vi "ZLIB VI Tree__ogtk.vi"() -> ()   [LabVIEW 2014]
uses:
  <userlib>/_OpenG.lib/lvzip/lvzip.llb/ZLIB File Info Old__ogtk.ctl
  <userlib>/_OpenG.lib/lvzip/lvzip.llb/ZLIB Compress File Info__ogtk.ctl
  <userlib>/_OpenG.lib/lvzip/lvzip.llb/ZLIB Uncompress File Info__ogtk.ctl
  <userlib>/_OpenG.lib/lvzip/lvzip.llb/ZLIB Unzip Handle__ogtk.ctl
  <userlib>/_OpenG.lib/lvzip/lvzip.llb/ZLIB Zip Handle__ogtk.ctl
  <userlib>/_OpenG.lib/lvzip/lvzip.llb/ZLIB File Info__ogtk.ctl
  <userlib>/_OpenG.lib/lvzip/lvzip.llb/ZLIB Open Zip Archive__ogtk.vi
  <userlib>/_OpenG.lib/lvzip/lvzip.llb/ZLIB Open Unzip Archive__ogtk.vi
  <userlib>/_OpenG.lib/lvzip/lvzip.llb/ZLIB Store File__ogtk.vi
  <userlib>/_OpenG.lib/lvzip/lvzip.llb/ZLIB Extract File__ogtk.vi
  <userlib>/_OpenG.lib/lvzip/lvzip.llb/ZLIB Open Unzip Stream__ogtk.vi
  <userlib>/_OpenG.lib/lvzip/lvzip.llb/ZLIB Store Stream__ogtk.vi
  <userlib>/_OpenG.lib/lvzip/lvzip.llb/ZLIB Extract Stream__ogtk.vi
panel:
  out "file info":T1 {"file timestamp" format="%<%H:%M:%S\n%d/%m/%Y>T"; "external fa" format="%.0x"; "internal fa" format="%.0x"; "crc" format="%.0x"}
  in  "zip file handle":T2
  in  "unzip file handle":T3
  out "unzip file info internal":T4 {"external fa" format="%.0x"; "internal fa" format="%.0x"; "crc" format="%.0x"}
  out "zip file info internal":T5
  out "file info old":T6 {"file timestamp" format="%<%H:%M:%S\n%d/%m/%Y>T"; "external fa" format="%.0x"; "internal fa" format="%.0x"; "crc" format="%.0x"}
  # "ZIP file library using the open source zlib library code with extension from Gilles Vollant.\nIn order to create a multi platform LabVIEW VI library some minor modification have been\nmade to the zlib library and ZIP file extension. The exported functions are all declared as\n__cdecl since this is the only platform independant calling convention available on all\nLabVIEW platforms. Doing it in this way allows us to use only one VI library which imports\nthe according shared library module, instead of having to maintain different VI libraries\nonly for the sake of different calling conventions.\nBecause of this and in order to avoid any incompatibilities with existing zlib libraries the\nshared library module has also been renamed to lvzlib.dll/so/cfr."
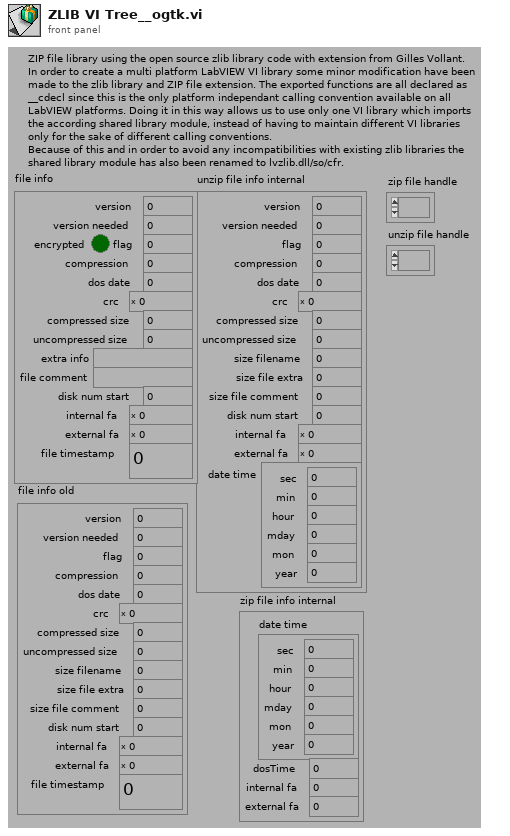
[diagram p1: front panel]
types:
  T1 = typedef "ZLIB File Info__ogtk.ctl" = cluster{"version":u32, "version needed":u32, "encrypted":bool, "flag":u32, "compression":i32, "dos date":u32, "crc":u32, "compressed size":u32, "uncompressed size":u32, "extra info":string, "file comment":string, "disk num start":u32, "internal fa":u32, "external fa":u32, "file timestamp":u32}
  T2 = typedef "ZLIB Zip Handle__ogtk.ctl" = refnum<k1>
  T3 = typedef "ZLIB Unzip Handle__ogtk.ctl" = refnum<k1>
  T4 = typedef "ZLIB Uncompress File Info__ogtk.ctl" = cluster{"version":u32, "version needed":u32, "flag":u32, "compression":u32, "dos date":u32, "crc":u32, "compressed size":u32, "uncompressed size":u32, "size filename":u32, "size file extra":u32, "size file comment":u32, "disk num start":u32, "internal fa":u32, "external fa":u32, "date time":cluster{"sec":i32, "min":i32, "hour":i32, "mday":i32, "mon":i32, "year":i32}}
  T5 = typedef "ZLIB Compress File Info__ogtk.ctl" = cluster{"date time":cluster{"sec":i32, "min":i32, "hour":i32, "mday":i32, "mon":i32, "year":i32}, "dosTime":u32, "internal fa":u32, "external fa":u32}
  T6 = typedef "ZLIB File Info Old__ogtk.ctl" = cluster{"version":u32, "version needed":u32, "flag":u32, "compression":u32, "dos date":u32, "crc":u32, "compressed size":u32, "uncompressed size":u32, "size filename":u32, "size file extra":u32, "size file comment":u32, "disk num start":u32, "internal fa":u32, "external fa":u32, "file timestamp":u32}
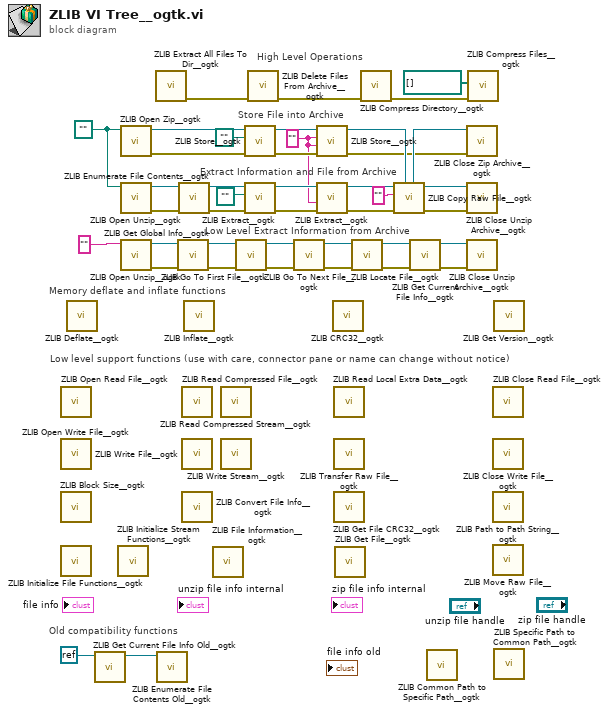
[diagram p0: block diagram]
diagram:
  w1 = ""
  w11 = path "" ("archive name")
  # "High Level Operations"
  # "Low level support functions (use with care, connector pane or name can change without notice)"
  # "Memory deflate and inflate functions"
  # "Old compatibility functions"
  # "Low Level Extract Information from Archive"
  # "Extract Information and File from Archive"
  # "Store File into Archive"
  n1 = call <userlib>:"ZLIB Open Read File__ogtk.vi"() -> ()  [unwired: 6 in, 4 out]
  n2 = call <userlib>:"ZLIB Open Write File__ogtk.vi"() -> ()  [unwired: 10 in, 2 out]
  n3 = call <userlib>:"ZLIB Block Size__ogtk.vi"() -> ()  [unwired: 2 in, 2 out]
  n4 = call <userlib>:"ZLIB Initialize File Functions__ogtk.vi"() -> ()  [unwired: 6 in, 2 out]
  n5 = call <userlib>:"ZLIB Deflate__ogtk.vi"() -> ()  [unwired: 5 in, 3 out]
  n6 = call <userlib>:"ZLIB Get Current File Info Old__ogtk.vi"("unzip Refnum"=refnum<k0> refnum) -> ("unzip Refnum out"=w21:T3)  [unwired: 3 in, 5 out]
  n7 = call <userlib>:"ZLIB Initialize Stream Functions__ogtk.vi"() -> ()  [unwired: 6 in, 2 out]
  n8 = call-poly <userlib>:"ZLIB Open Zip__ogtk.vi"("archive name"=w11) -> ("error out"=w30:errorcluster, "zip Refnum"=w31:T2)  [unwired: 4 in, 1 out]
  n9 = call-poly <userlib>:"ZLIB Open Unzip__ogtk.vi"("archive name"=w11) -> ("error out"=w23:errorcluster, "unzip Refnum"=w24:T3)  [unwired: 5 in]
  n10 = call-poly <userlib>:"ZLIB Open Unzip__ogtk.vi"("archive stream"="") -> ("error out"=w28:errorcluster, "unzip Refnum"=w29:T3)  [unwired: 5 in]
  n11 = call <userlib>:"ZLIB Extract All Files To Dir__ogtk.vi"() -> ("error out"=w18:errorcluster)  [unwired: 9 in, 2 out]
  n12 = call <userlib>:"ZLIB Enumerate File Contents Old__ogtk.vi"("unzip Refnum"=w21) -> ()  [unwired: 4 in, 7 out]
  n13 = call <userlib>:"ZLIB Get Global Info__ogtk.vi"("error in (no error)"=w28, "unzip Refnum"=w29) -> ("error out"=w34:errorcluster, "unzip Refnum out"=w35:T3)  [unwired: 2 in, 2 out]
  n14 = call <userlib>:"ZLIB Enumerate File Contents__ogtk.vi"("error in (no error)"=w23, "unzip Refnum"=w24) -> ("error out"=w26:errorcluster, "unzip Refnum out"=w27:T3)  [unwired: 5 in, 3 out]
  n15 = call <userlib>:"ZLIB Read Compressed File__ogtk.vi"() -> ()  [unwired: 8 in, 2 out]
  n16 = call <userlib>:"ZLIB Write File__ogtk.vi"() -> ()  [unwired: 7 in, 2 out]
  n17 = call <userlib>:"ZLIB Convert File Info__ogtk.vi"() -> ()  [unwired: 3 in, 1 out]
  n18 = call <userlib>:"ZLIB Inflate__ogtk.vi"() -> ()  [unwired: 5 in, 3 out]
  n19 = call <userlib>:"ZLIB File Information__ogtk.vi"() -> ()  [unwired: 4 in, 6 out]
  n20 = call <userlib>:"ZLIB Read Compressed Stream__ogtk.vi"() -> ()  [unwired: 7 in, 3 out]
  n21 = call <userlib>:"ZLIB Write Stream__ogtk.vi"() -> ()  [unwired: 7 in, 2 out]
  n22 = call <userlib>:"ZLIB Go To First File__ogtk.vi"("error in (no error)"=w34, "unzip Refnum"=w35) -> ("error out"=w40:errorcluster, "unzip Refnum out"=w41:T3)  [unwired: 4 in]
  n23 = call-poly <userlib>:"ZLIB Store__ogtk.vi"("error in (no error)"=w30, "source path"=path "", "zip Refnum"=w31) -> ("error out"=w5:errorcluster, "zip Refnum out"=w4:T2)  [unwired: 7 in]
  n24 = call-poly <userlib>:"ZLIB Extract__ogtk.vi"("error in (no error)"=w26, "target path"=path "", "unzip Refnum"=w27) -> ("error out"=w9:errorcluster, "unzip Refnum out"=w8:T3)  [unwired: 5 in]
  n25 = call <userlib>:"ZLIB Delete Files From Archive__ogtk.vi"("error in (no error)"=w18) -> ("error out"=w17:errorcluster)  [unwired: 9 in, 1 out]
  n26 = call <userlib>:"ZLIB Go To Next File__ogtk.vi"("error in (no error)"=w40, "unzip Refnum"=w41) -> ("error out"=w38:errorcluster, "unzip Refnum out"=w39:T3)  [unwired: 4 in]
  n27 = call-poly <userlib>:"ZLIB Store__ogtk.vi"("error in (no error)"=w5, "internal name"=w1, "source stream"=w1, "zip Refnum"=w4) -> ("error out"=w2:errorcluster, "zip Refnum out"=w3:T2)  [unwired: 6 in]
  n28 = call-poly <userlib>:"ZLIB Extract__ogtk.vi"("error in (no error)"=w9, "internal name"=w1, "unzip Refnum"=w8) -> ("error out"=w6:errorcluster, "unzip Refnum out"=w7:T3)  [unwired: 4 in, 1 out]
  n29 = call <userlib>:"ZLIB CRC32__ogtk.vi"() -> ()  [unwired: 6 in, 2 out]
  n30 = call <userlib>:"ZLIB Read Local Extra Data__ogtk.vi"() -> ()  [unwired: 5 in, 3 out]
  n31 = call <userlib>:"ZLIB Transfer Raw File__ogtk.vi"() -> ()  [unwired: 6 in, 3 out]
  n32 = call <userlib>:"ZLIB Get File CRC32__ogtk.vi"() -> ()  [unwired: 6 in, 2 out]
  n33 = call <userlib>:"ZLIB Get File__ogtk.vi"() -> ()  [unwired: 8 in, 2 out]
  n34 = call <userlib>:"ZLIB Locate File__ogtk.vi"("error in (no error)"=w38, "unzip Refnum"=w39) -> ("error out"=w37:errorcluster, "unzip Refnum out"=w36:T3)  [unwired: 4 in]
  n35 = call <userlib>:"ZLIB Compress Directory__ogtk.vi"("error in (no error)"=w17) -> ("error out"=w16:errorcluster)  [unwired: 8 in, 2 out]
  n36 = call <userlib>:"ZLIB Copy Raw File__ogtk.vi"("zip Refnum"=w3, "error in (no error)"=w6, "name (empty: use current)"="" ("name"), "unzip Refnum"=w7) -> ("error out"=w19:errorcluster, "unzip Refnum out"=w20:T3, "zip Refnum out"=w13:T2)  [unwired: 5 in]
  n37 = call <userlib>:"ZLIB Get Current File Info__ogtk.vi"("error in (no error)"=w37, "unzip Refnum"=w36) -> ("error out"=w32:errorcluster, "unzip Refnum out"=w33:T3)  [unwired: 6 in, 2 out]
  n38 = call <userlib>:"ZLIB Common Path to Specific Path__ogtk.vi"() -> ()  [unwired: 11 in, 1 out]
  n39 = call <userlib>:"ZLIB Close Zip Archive__ogtk.vi"("error in (no error)"=w2, "zip Refnum"=w13) -> ()  [unwired: 4 in, 2 out]
  n40 = call <userlib>:"ZLIB Close Unzip Archive__ogtk.vi"("error in (no error)"=w19, "unzip Refnum"=w20) -> ()  [unwired: 5 in, 1 out]
  n41 = call <userlib>:"ZLIB Close Unzip Archive__ogtk.vi"("error in (no error)"=w32, "unzip Refnum"=w33) -> ()  [unwired: 5 in, 1 out]
  n42 = call <userlib>:"ZLIB Compress Files__ogtk.vi"("error in (no error)"=w16, "file names"=path[] []) -> ()  [unwired: 8 in, 2 out]
  n43 = call <userlib>:"ZLIB Close Read File__ogtk.vi"() -> ()  [unwired: 10 in, 2 out]
  n44 = call <userlib>:"ZLIB Close Write File__ogtk.vi"() -> ()  [unwired: 6 in, 2 out]
  n45 = call <userlib>:"ZLIB Path to Path String__ogtk.vi"() -> ()  [unwired: 6 in, 2 out]
  n46 = call <userlib>:"ZLIB Move Raw File__ogtk.vi"() -> ()  [unwired: 9 in, 3 out]
  n47 = call <userlib>:"ZLIB Get Version__ogtk.vi"() -> ()  [unwired: 1 out]
  n48 = call <userlib>:"ZLIB Specific Path to Common Path__ogtk.vi"() -> ()  [unwired: 11 in, 1 out]
